vi "cm_Launch Reentrant VI.vi"(8 "error in (no error)":errorcluster, 9 "Initial Message Values":string[](array[string]), 10 "Initial Message Names":string[](array[string]), 11 "VI path":path) -> (0 "error out":errorcluster, 3 "VI Refnum":refnum<vi>)   [LabVIEW 2012, in "Channel Monitor.xctl"]
uses:
  Channel Monitor.xctl
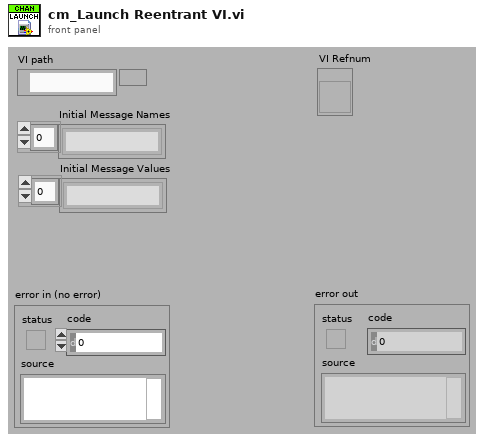
[diagram p1: front panel]
types:
  T1 = typedef "amc_Message Queue.ctl" = refnum<queue>
  T2 = enum32{"Bad", "Idle", "Run top level", "Running"}
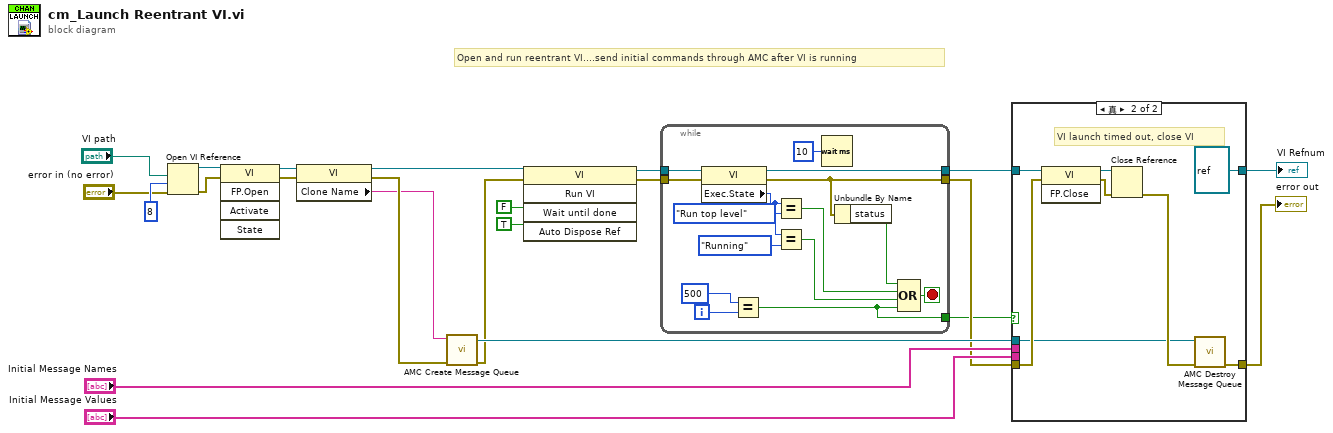
[diagram p0: block diagram]
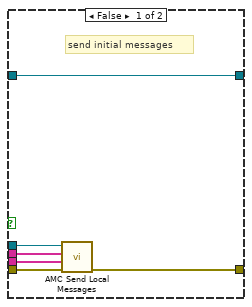
[diagram p2: hidden frame]
diagram:
  # "Open and run reentrant VI....send initial commands through AMC after VI is running"
  n1 = Open VI Reference(vi path="VI path", options=8, error in (no error)="error in (no error)") -> (vi reference=w19:refnum<vi>, error out=w18:errorcluster)  [unwired: 3 in]
  n2 = invoke class="VI" method="FP.Open"(reference=w19, error in=w18) -> (reference out=w17:refnum<vi>, error out=w16:errorcluster)  [unwired: 3 in, 3 out]
  n3 = property class="VI"(reference=w17, error in=w16) -> (reference out=w15:refnum<vi>, error out=w13:errorcluster, "Clone Name"=w1:string)
  n4 = call <userlib>:"AMC Create Message Queue.vi"("error in (no error)"=w13, "Message Queue Name"=w1) -> ("error out"=w8:errorcluster, "Message Queue out"=w12:T1)  [unwired: 2 in, 6 out]
  n5 = invoke class="VI" method="Run VI"(reference=w15, error in=w8, "Wait until done"=FALSE ("Wait Until Done"), "Auto Dispose Ref"=TRUE ("Auto Dispose Reference")) -> (reference out=w9:refnum<vi>, error out=w6:errorcluster)  [unwired: 1 in, 3 out]
  n6 = while {
    tunnel: w9 -> [w38]
    tunnel: [w37] -> w3
    tunnel: [w36] -> w7
    tunnel: w6 -> [w30]
    tunnel: [w25] -> w5
    i -> [w24]
    stop <- w33 stop-if-true
    n7 = property class="VI"(reference=w38, error in=w30) -> (reference out=w37:refnum<vi>, error out=w36:errorcluster, "Exec.State"=w28:T2)
    n8 = Equal?(x=500, y=w24) -> (x = y?=w25:bool)
    n9 = Equal?(x=w28, y=T2."Run top level" ("Execution:State")) -> (x = y?=w29:bool)
    n10 = Equal?(x=w28, y=T2."Running" ("Execution:State")) -> (x = y?=w26:bool)
    n11 = Wait (ms)(milliseconds to wait=u32 10) -> ()  [unwired: 1 out]
    n12 = Unbundle By Name(w36) -> ("status"=w34:bool)
    n13 = Compound Arithmetic op=OR(w34, w29, w26, w25) -> (w33:bool)
  }
  n14 = case shown="真" w5 {
    tunnel: w12 -> [w44 w45]
    tunnel: "Initial Message Names" -> [w43 _]
    tunnel: "Initial Message Values" -> [w42 _]
    tunnel: w7 -> [w41 w49]
    tunnel: [w40 w47] -> w4
    tunnel: w3 -> [w39 w52]
    tunnel: [w39 refnum<vi> refnum] -> w2
    frame False {
      # "send initial messages"
      n15 = call <userlib>:"AMC Send Local Messages.vi"("error in (no error)"=w41, "Message Values"=w42, "Message Names"=w43, "Message Queue in"=w44) -> ("error out"=w40:errorcluster)  [unwired: 6 in, 1 out]
    }
    frame True {
      # "VI launch timed out, close VI"
      n16 = invoke class="VI" method="FP.Close"(reference=w52, error in=w49) -> (reference out=w51:refnum<vi>, error out=w48:errorcluster)  [unwired: 1 in, 1 out]
      n17 = Close Reference(reference=w51, error in (no error)=w48) -> (error out=w46:errorcluster)
      n18 = call <userlib>:"AMC Destroy Message Queue.vi"("error in (no error)"=w46, "Message Queue in"=w45) -> ("error out"=w47:errorcluster)  [unwired: 8 in, 1 out]
    }
  }
  "VI Refnum" <- w2
  "error out" <- w4
